vi "GetParam.vi"(8 "error in (no error)":errorcluster caption="entrée d'erreur (pas d'erreur)", 11 "Silhouette_Score.lvclass":refnum<class "Silhouette_Score.lvclass">) -> (0 "error out":errorcluster caption="sortie d'erreur", 2 "silhouette_score":T1={"metric"="euclidean", "sample_size"="", "random_state"=0} {"random_state" min=-1}, 3 "Silhouette_Score.lvclass":refnum<class "Silhouette_Score.lvclass">)   [LabVIEW 2020, in "Silhouette_Score.lvclass"]
doc: "Get Parameters"
uses:
  Silhouette_Score.lvclass
  Silhouette_Score.lvclass/Silhouette_Score.ctl
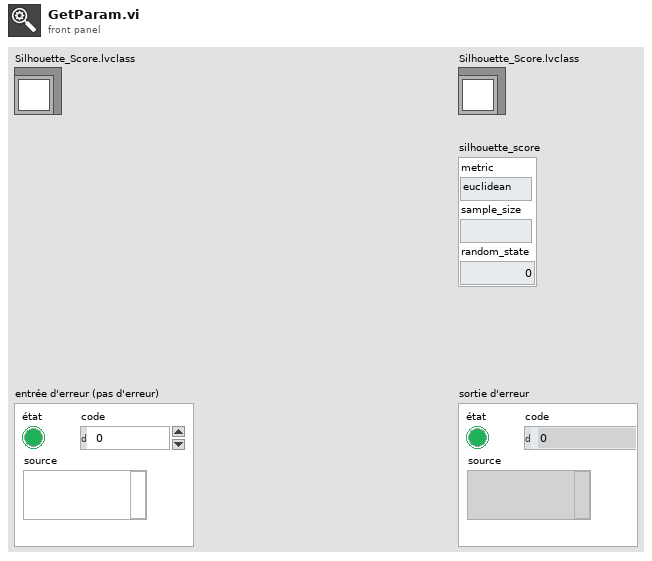
[diagram p1: front panel]
types:
  T1 = cluster{"metric":string, "sample_size":string, "random_state":i32}
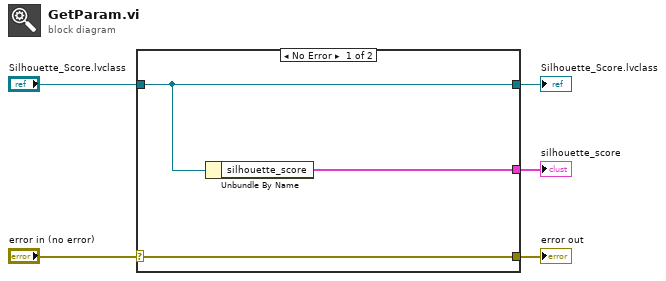
[diagram p0: block diagram]
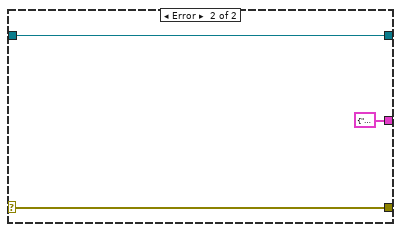
[diagram p2: hidden frame]
diagram:
  n1 = case shown="No Error" "error in (no error)" {
    selector: "error in (no error)" -> [w8 w10]
    tunnel: [w8 w10] -> w4
    tunnel: [w7 w11] -> w2
    tunnel: "Silhouette_Score.lvclass" -> [w7 w11]
    tunnel: [w6 T1 {"metric"="", "sample_size"="", "random_state"=0} ("silhouette_score")] -> w1
    frame No Error {
      n2 = Unbundle By Name(w7) -> ("silhouette_score"=w6:T1)
    }
    frame Error {
    }
  }
  "error out" <- w4
  "Silhouette_Score.lvclass" <- w2
  "silhouette_score" <- w1
